vi "Read Pots.vi"() -> (0 "Pot Write Cluster":T1, 2 "Right Pot":dbl, 3 "Left Pot":dbl, 4 "Unzeroed Right Pot":dbl, 6 "Unzeroed Left Pot":dbl)   [LabVIEW 2015]
uses:
  Pot Data.ctl
  Robot Global Data.vi
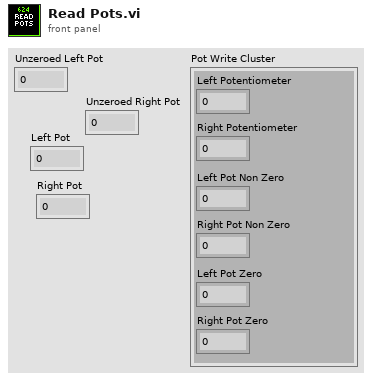
[diagram p1: front panel]
types:
  T1 = typedef "Pot Data.ctl" = cluster{"Left Pot Zero":sgl, "Right Pot Zero":sgl, "Left Potentiometer":sgl, "Right Potentiometer":sgl, "Left Pot Non Zero":sgl, "Right Pot Non Zero":sgl}
  T2 = typedef "Dashboard Control Data.ctl" = cluster{"Cam Exposure":dbl, "Go to angle":dbl, "Steer PID Gains":cluster{"proportional gain (Kc)":dbl, "integral time (Ti, min)":dbl, "derivative time (Td, min)":dbl}, "Steer PID output Range":cluster{"output high":dbl, "output low":dbl}, "Pressure m \nValue":dbl, "Pressure b \nValue":dbl, "Roller Command Cluster ":T3, "Elevator":T4, "Encoder Control":T6, "Auton Settings":cluster{"Drive Dist Window Size":dbl}, "Drivetrain Settings":T7, "Lance":T8}
  T3 = typedef "Roller Control.ctl" = cluster{"Intake Speed":dbl, "Turn In Speed":dbl, "Unload Speed":dbl, "Turn Out Speed":dbl, "Ping Align Tolerance":dbl, "Tote Range Threshold":dbl, "Right Pot 0":dbl, "Pot Threshold":dbl, "Left Pot 0":dbl, "Right Pot Scale":dbl, "Left Pot Scale":dbl, "Min Elevator Height":dbl, "Eject Time":dbl, "Eject US Threshold":dbl, "Anti-Twitch Time":u32, "Ping Caring Threshold":dbl, "Pot Diff Threshold":dbl, "Pinch Sustain":u32, "Absorb Give Up Threshold":dbl, "Untip In Threshold":dbl, "Untip Grab Range":dbl, "Ultrasonic Hold Time":u32, "Landscape Absorb Time":u32, "Pot Use Wait Time":u32, "Can Turn Stop Range":dbl, "HP Load Speed":dbl, "Stick Multiplier":dbl, "Coop Eject Speed":dbl}
  T4 = typedef "Elevator DB Control.ctl" = cluster{"PID Output Range":cluster{"output high":dbl, "output low":dbl}, "PID gains":cluster{"proportional gain (Kc)":dbl, "integral time (Ti, min)":dbl, "derivative time (Td, min)":dbl}, "Height Tolerance":sgl, " Encoder Constant":dbl, "Eject Time":sgl, "Zeroing Speed":sgl, "Presets":T5, "Ping Detect Threshold":sgl, "Trashcan Detect Threshold":sgl, "Zero Filter Time":dbl, "Stabilizer Open Time":dbl, "Zero Creep Speed":dbl, "Max Current":dbl, "Current Trip Time":dbl, "Abort Pitch":dbl, "Finger m":dbl, "Finger b":dbl, "Finger max ":dbl, "Finger Stabilizer":dbl, "Finger Store":dbl, "Finger Stop Store":dbl, "Stabilizer Close Time":dbl, "Finger min":dbl, "Unstick gain":dbl, "Full Detect Max":dbl}
  T5 = typedef "Elevator Presets.ctl" = cluster{"Pickup 2 w/ Tote":sgl, "Pickup 2 w/ Trashcan":sgl, "Pickup 3 w/ Tote":sgl, "Pickup 3 w/ Trashcan":sgl, "Bottom":sgl, "Pickup 1 w/ Tote":sgl, "Pickup Trashcan":sgl, "Pickup 1 w/ Trashcan":sgl, "Eject":sgl, "Hold Low":sgl, "Step add height":sgl, "Untip Lift":dbl, "Drop Stack":dbl, "HP Load Hold":dbl, "HP Load Drop":dbl, "HP Load Hold Can":dbl, "Store can max":dbl, "HP Drag Score":dbl, "HP Drag Finish":dbl, "Finger trashcan avoid":dbl, "Full":dbl}
  T6 = typedef "Encoder Control.ctl" = cluster{"Left Tick Constant":dbl, "Right Tick Constant":dbl, "Center Tick Constant":dbl, "Reset?":bool, "Y Dist":cluster{"PID gains":cluster{"proportional gain (Kc)":dbl, "integral time (Ti, min)":dbl, "derivative time (Td, min)":dbl}}, "X Dist":cluster{"PID gains":cluster{"proportional gain (Kc)":dbl, "integral time (Ti, min)":dbl, "derivative time (Td, min)":dbl}}, "Y Stop Thresh":dbl, "Y Stop Speed":dbl, "X Stop Thresh":dbl, "X Stop Speed":dbl}
  T7 = typedef "Drivetrain Settings.ctl" = cluster{"Gyro Tolerance":sgl, "Strafe Correct max steer":sgl, "Strafe Timer Wait":sgl, "Throttle Ramp (ms)":sgl, "Strafe Ramp (ms)":sgl, "Angular rate compensation":bool, "Throttle to Rate Scale":sgl, "Rate compensation gain":sgl, "Creep Steer":sgl, "Creep Throttle":sgl}
  T8 = typedef "Pike DB Controls.ctl" = cluster{"Down Speed":dbl, "Up Speed":dbl, "Max Down Time":dbl, "Max Up Time":dbl, "Current Limit":dbl}
  T9 = typedef "WPI_PotentiometerDevRef.ctl" = cluster{"DevStatus":errorcluster, "Analog Channel":T10, "Invert Output":bool}
  T10 = typedef "FPGA_AIChannel.ctl" = enum8{"AI 0", "AI 1", "AI 2", "AI 3", "AI MXP 0", "AI MXP 1", "AI MXP 2", "AI MXP 3", "Invalid"}
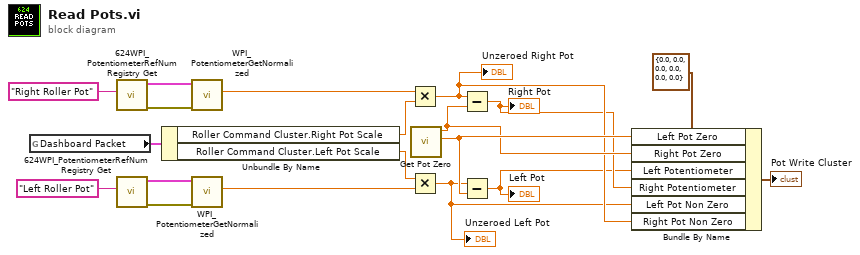
[diagram p0: block diagram]
diagram:
  n1 = global read "Robot Global Data.vi" "Dashboard Packet"() -> (w13:T2)
  n2 = call "624WPI_PotentiometerRefNum Registry Get.vi"("refnum name"="Right Roller Pot") -> ("error out"=w19:errorcluster, "PotDevRef"=w18:T9)  [unwired: 9 in]
  n3 = call "624WPI_PotentiometerRefNum Registry Get.vi"("refnum name"="Left Roller Pot") -> ("error out"=w16:errorcluster, "PotDevRef"=w17:T9)  [unwired: 9 in]
  n4 = Unbundle By Name(w13) -> ("Roller Command Cluster.Right Pot Scale"=w10:dbl, "Roller Command Cluster.Left Pot Scale"=w9:dbl)
  n5 = call <vilib>:"WPI_PotentiometerGetNormalized.vi"("error in"=w19, "PotDevRef"=w18) -> ("Normalized Value"=w12:dbl)  [unwired: 7 in, 2 out]
  n6 = call <vilib>:"WPI_PotentiometerGetNormalized.vi"("error in"=w16, "PotDevRef"=w17) -> ("Normalized Value"=w11:dbl)  [unwired: 7 in, 2 out]
  n7 = Multiply(x=w12, y=w10) -> (x*y=w5:dbl)
  "Unzeroed Right Pot" <- w5
  n8 = Multiply(x=w9, y=w11) -> (x*y=w4:dbl)
  "Unzeroed Left Pot" <- w4
  n9 = call "Get Pot Zero.vi"() -> ("Left Pot 0"=w7:dbl, "Right Pot 0"=w6:dbl)  [unwired: 10 in]
  n10 = Subtract(x=w5, y=w6) -> (x-y=w3:dbl)
  "Right Pot" <- w3
  n11 = Subtract(x=w4, y=w7) -> (x-y=w2:dbl)
  "Left Pot" <- w2
  n12 = Bundle By Name(cluster=T1 {"Left Pot Zero"=0.0, "Right Pot Zero"=0.0, "Left Potentiometer"=0.0, "Right Potentiometer"=0.0, "Left Pot Non Zero"=0.0, "Right Pot Non Zero"=0.0} ("Potentiometer Cluster"), "Left Pot Zero"=w7, "Right Pot Zero"=w6, "Left Potentiometer"=w2, "Right Potentiometer"=w3, "Left Pot Non Zero"=w4, "Right Pot Non Zero"=w5) -> (→"Pot Write Cluster":T1)
